vi "SendMessage.vi"(8 "error in (no error)":errorcluster, 9 "Data":variant, 10 "Command":string, 11 "JQMHStartup in":refnum<class "JQMHStartup.lvclass">) -> (0 "error out":errorcluster, 3 "JQMHStartup out":refnum<class "JQMHStartup.lvclass">)   [LabVIEW 2024, in "JQMHStartup.lvclass"]
uses:
  JQMHStartup.lvclass
  JQMHStartup.lvclass/JQMHStartup.ctl
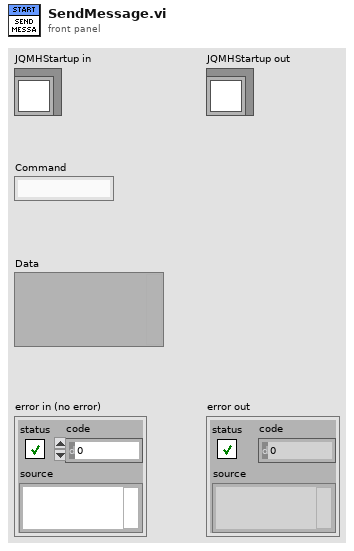
[diagram p1: front panel]
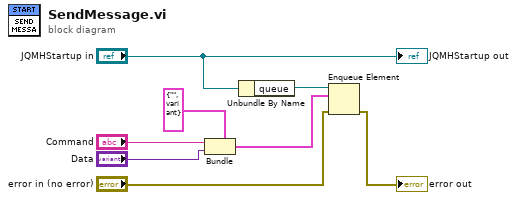
[diagram p0: block diagram]
diagram:
  n1 = Bundle(cluster=cluster{string, variant} {"", variant} ("element"), "Command", "Data") -> (w1:cluster{string, variant})
  n2 = Unbundle By Name("JQMHStartup in") -> ("queue"=w5:refnum<queue>)
  n3 = Enqueue Element(queue=w5, element=w1, error in (no error)="error in (no error)") -> (error out=→"error out":errorcluster)  [unwired: 1 in, 2 out]
  "JQMHStartup out" <- "JQMHStartup in"
